vi "Write Specific Mode Class.vi"(8 "error in (no error)":errorcluster, 10 "Communication.lvclass":refnum<class "Communication.lvclass">, 11 "Sender in":refnum<class "Sender.lvclass">) -> (0 "error out":errorcluster, 3 "Sender out":refnum<class "Sender.lvclass">)   [LabVIEW 2023, in "Sender.lvclass"]
uses:
  Sender.lvclass
  Sender.lvclass/Sender.ctl
  Communication/Communication.lvclass
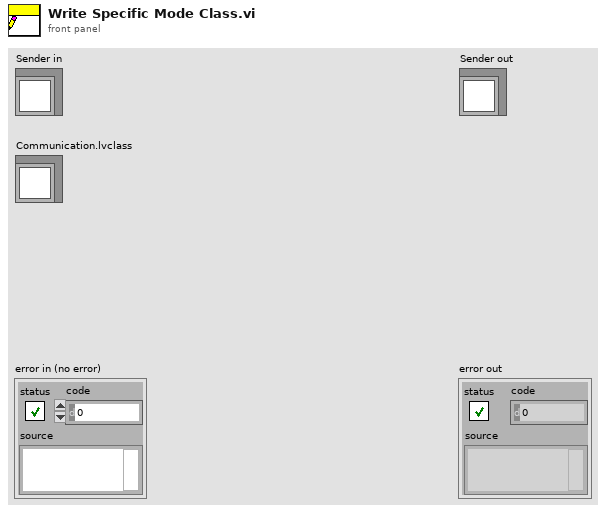
[diagram p1: front panel]
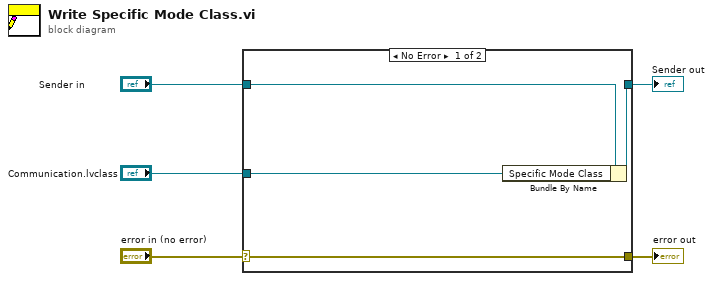
[diagram p0: block diagram]
diagram:
  n1 = case shown="No Error" "error in (no error)" {
    selector: "error in (no error)" -> [w9 w10]
    tunnel: [w9 w10] -> w4
    tunnel: [w7 w11] -> w2
    tunnel: "Sender in" -> [w8 w11]
    tunnel: "Communication.lvclass" -> [w6 _]
    frame No Error {
      n2 = Bundle By Name(cluster=w8, "Specific Mode Class"=w6) -> (w7:refnum<class "Sender.lvclass">)
    }
    frame Error {
    }
  }
  "error out" <- w4
  "Sender out" <- w2
